vi "TF_analyse.vi"(0 "image 2D":dbl[][](array[numeric]), 7 "FLUENCE calculation":bool) -> (20 "position max en x":i32, 21 "position max en y":i32, 22 "FWHM en x":dbl, 23 "FWHM en y":dbl, 24 "coupes x & y":dbl[][](array[numeric]), 25 "valeur max":dbl, 27 "intégration totale":dbl caption="image intégrée\nnormalisée")   [LabVIEW 2014]
uses:
  <vilib>/Analysis/2dsp.llb/Integral Method.ctl
  <vilib>/Analysis/8numeric.llb/2D Numeric Integration.vi
  <vilib>/Analysis/NI_AALPro.lvlib
panel:
  # "SORTIES"
  # "ENTREES"
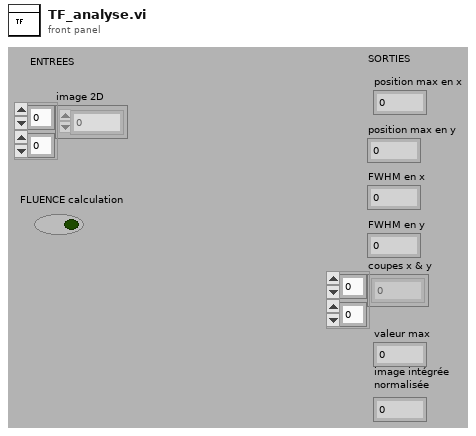
[diagram p1: front panel]
types:
  T1 = typedef "NI_AALPro.lvlib/Integral Method.ctl" = i32
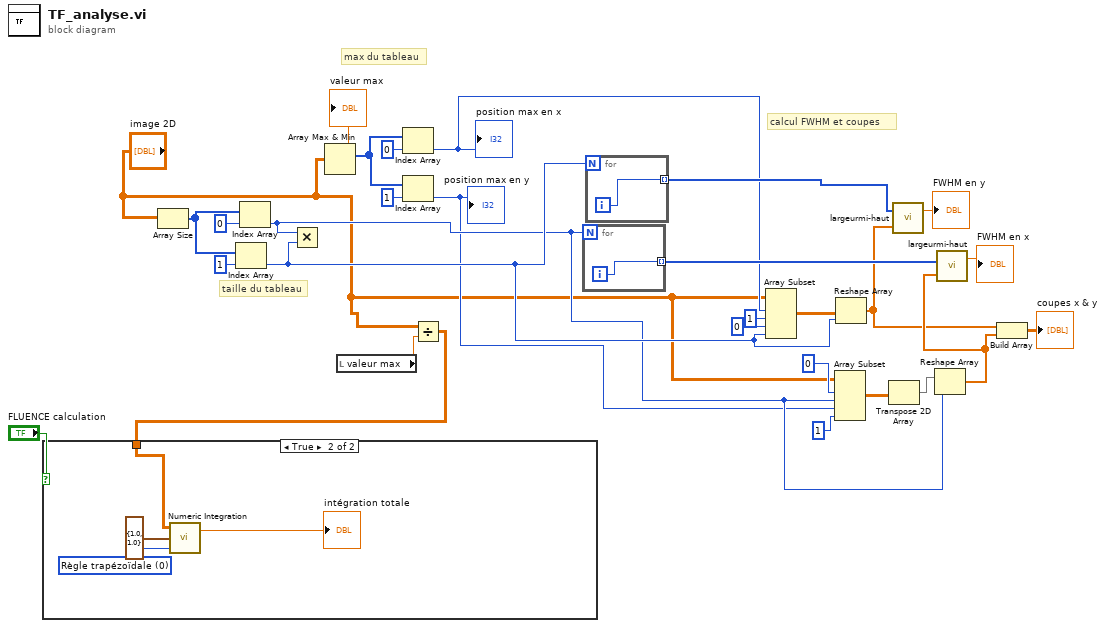
[diagram p0: block diagram]
diagram:
  # "calcul FWHM et coupes"
  # "max du tableau"
  # "taille du tableau"
  n1 = Array Size(array="image 2D") -> (size(s)=w24:i32[])
  n2 = Index Array(array=w24, index=1 ("indice")) -> (element=w9:i32)
  n3 = Index Array(array=w24, index=0 ("indice")) -> (element=w8:i32)
  n4 = Multiply(x=w8, y=w9) -> ()  [unwired: 1 out]
  n5 = Array Max & Min(array="image 2D") -> (max value=→"valeur max":dbl, max index (indices)=w27:i32[])  [unwired: 2 out]
  n6 = local read "valeur max"() -> (w3:dbl)
  n7 = Index Array(array=w27, index=0 ("indice")) -> (element=w7:i32)
  "position max en x" <- w7
  n8 = Index Array(array=w27, index=1 ("indice")) -> (element=w6:i32)
  "position max en y" <- w6
  n9 = Divide(x="image 2D", y=w3) -> (x/y=w2:dbl[][])
  n10 = case shown="True" "FLUENCE calculation" {
    tunnel: w2 -> [_ w31]
    frame False {
    }
    frame True {
      w32 = T1 0 items=["Règle trapézoïdale", "Règle de Simpson", "Règle de Simpson 3/8", "Règle de Bode"] ("integration method")
      n11 = call-poly <vilib>:"Numeric Integration.vi"("integration method"=w32, "interval size"=cluster{"dx":dbl, "dy":dbl} {"dx"=1.0, "dy"=1.0}, "Input Array"=w31) -> ("result"=→"intégration totale":dbl)  [unwired: 1 out]
    }
  }
  n12 = for {
    N: w8 -> [_]
    tunnel: [w34] -> w13 mode=indexing
    i -> [w34]
  }
  n13 = for {
    N: w9 -> [_]
    tunnel: [w35] -> w14 mode=indexing
    i -> [w35]
  }
  n14 = Array Subset(array="image 2D", index (row)=w7, length (row)=1 ("longueur"), index (col)=0 ("indice"), length (col)=w9) -> (w18:dbl[][])
  n15 = Array Subset(array="image 2D", index (row)=0 ("indice"), length (row)=w8, index (col)=w6, length (col)=1 ("longueur")) -> (w19:dbl[][])
  n16 = Reshape Array(w18, w9) -> (w12:dbl[])
  n17 = Transpose 2D Array(2D array=w19) -> (transposed array=w17:dbl[][])
  n18 = call "largeurmi-haut.vi"("Y"=w12, "X"=w14) -> ("FWHM"=→"FWHM en y":dbl)  [unwired: 1 in]
  n19 = Reshape Array(w17, w8) -> (w16:dbl[])
  n20 = call "largeurmi-haut.vi"("Y"=w16, "X"=w13) -> ("FWHM"=→"FWHM en x":dbl)  [unwired: 1 in]
  n21 = Build Array(w12, w16) -> (→"coupes x & y":dbl[][])
